vi "Get Column Configuration.vi"(8 "error in (no error)":errorcluster, 11 "Composed Column in":refnum<class "Composed Column.lvclass">) -> (0 "error out":errorcluster, 2 "Column Configuration":refnum<class "Column Configuration.lvclass">, 3 "Composed Column out":refnum<class "Composed Column.lvclass">)   [LabVIEW 2020, in "Composed Columns.lvlib" / "Composed Column.lvclass"]
uses:
  Composed Column.lvclass
  Basic Columns/Column Configuration/Basic Column Configuration Class/Column Configuration.lvclass
  Composed Column.lvclass/Composed Column.ctl
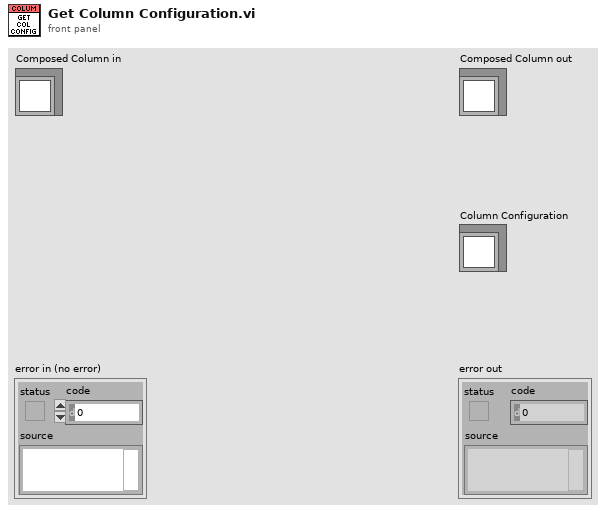
[diagram p1: front panel]
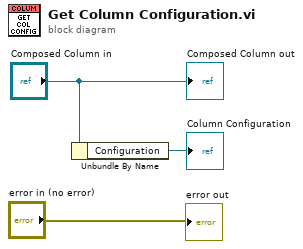
[diagram p0: block diagram]
diagram:
  n1 = Unbundle By Name("Composed Column in") -> ("Configuration"=→"Column Configuration":refnum<class "Column Configuration.lvclass">)
  "error out" <- "error in (no error)"
  "Composed Column out" <- "Composed Column in"
